vi "Begin.vi"(8 "error in":errorcluster) -> (0 "error out":errorcluster)   [LabVIEW 2016]
doc: "Called before other user functions, this VI is expected to open initial I/O refnums, load in file data, and do all program initialization. Notice that the <B>error out</B> terminal is simply used for data flow. Wiring it to other structures or subVIs ensures that this VI runs first."
uses:
  <vilib>/Rock Robotics/SystemInterfaces/spilib/spi_bus.ctl
  <vilib>/Rock Robotics/WPI/SPI/WPI_SPIMode.ctl
  <vilib>/Rock Robotics/SystemInterfaces/DIO/FPGA_DIOPWMChannel.ctl
  <vilib>/Rock Robotics/WPI/SafetyOutput/WPI_SafetyOutputConfigMenu.ctl
  <vilib>/Rock Robotics/WPI/DriverStation/WPI_DriverStationRobotMode2.ctl
  <vilib>/Rock Robotics/WPI/Joystick/WPI_JoystickDeviceEnum.ctl
  <vilib>/Rock Robotics/SystemInterfaces/DIO/FPGA_DIOChannel.ctl
  <vilib>/Rock Robotics/WPI/Encoder/WPI_EncoderType.ctl
  NI WPI/WPI_SerialPort_USB.ctl
  <vilib>/Rock Robotics/WPI/ThirdParty/CanMotor/TalonSRX/WPI_CANTalonSRX_APIControlMode.ctl
  <vilib>/Rock Robotics/WPI/Solenoid/WPI_SolenoidChannel.ctl
  <vilib>/Rock Robotics/SystemInterfaces/i2clib/i2c_bus.ctl
  <vilib>/Rock Robotics/WPI/Solenoid/WPI_SolenoidValue.ctl
  Robot Global Data.vi
  <vilib>/Rock Robotics/Network Tables/NT Write String Array.vi
  <vilib>/Rock Robotics/WPI/Counter/WPI_CounterDigitalInputToDigitalSource.vi
  navX Library v2/IO/Open/Z900_navX_Open_Serial.vi
  <vilib>/Rock Robotics/WPI/Solenoid/WPI_SolenoidOpenSingle.vi
  <vilib>/Rock Robotics/WPI/MotorControl/WPI_MotorControlOpen VictorSP.vi
  <vilib>/Rock Robotics/WPI/RobotDrive/WPI_RobotDriveOpen4MotorWithVictorSP.vi
  <vilib>/Rock Robotics/WPI/Solenoid/WPI_SolenoidSetEnum.vi
  navX Library v2/navX Library v2.lvlib
  NI WPI/NI WPI Serial USB.lvlib
panel:
  in  "Chip Select Active High (F)":bool
  in  "Mode (3)":T1=enum."Mode 3 (Clk Idle High,Sample on Trailing)"
  in  "Clock Rate (Hz)":dbl=500000.0
  in  "SPI Bus":T2=enum."SPI On-Board, CS1"
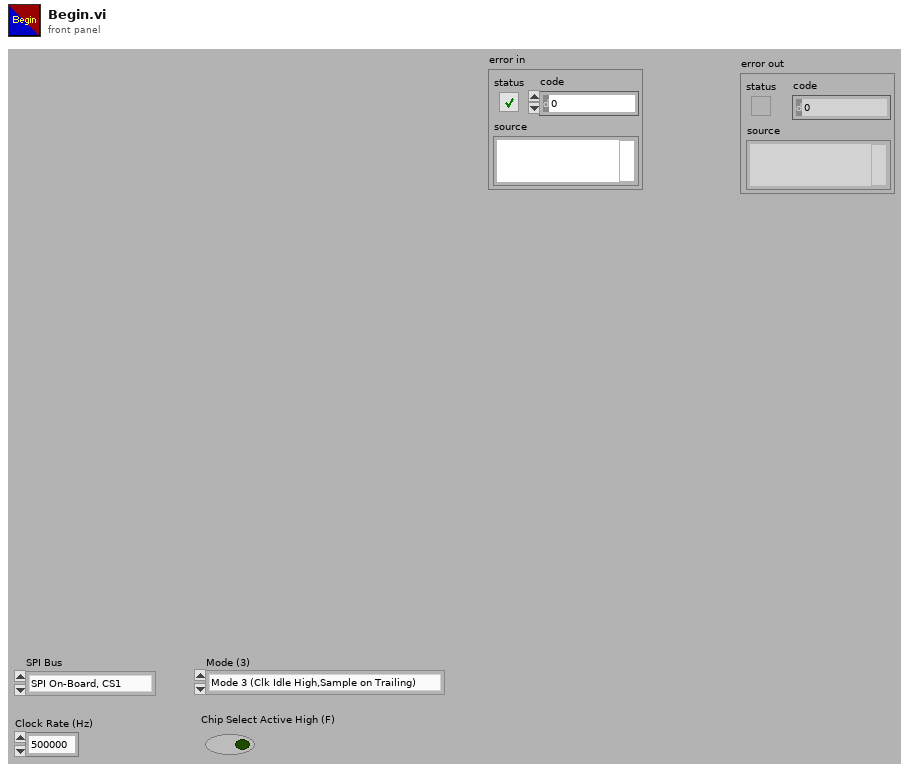
[diagram p1: front panel]
types:
  T1 = typedef "WPI_SPIMode.ctl" = enum16{"Mode 0 (Clk Idle Low,Sample on Leading)", "Mode 1 (Clk Idle Low,Sample on Trailing)", "Mode 2 (Clk Idle High,Sample on Leading)", "Mode 3 (Clk Idle High,Sample on Trailing)"}
  T2 = typedef "spi_bus.ctl" = enum16{"SPI On-Board, CS0", "SPI On-Board, CS1", "SPI On-Board, CS2", "SPI On-Board, CS3", "SPI MXP", "Invalid"}
  T3 = typedef "WPI_CANTalonSRX_APIControlMode.ctl" = enum8{"Percent VBus", "Speed", "Position", "Slave", "Unchanged / Invalid", "Voltage Compensation", "Current", "Motion Profile", "Motion Magic"}
  T4 = typedef "FPGA_DIOPWMChannel.ctl" = enum8{"PWM 0", "PWM 1", "PWM 2", "PWM 3", "PWM 4", "PWM 5", "PWM 6", "PWM 7", "PWM 8", "PWM 9", "PWM MXP 0", "PWM MXP 1", "PWM MXP 2", "PWM MXP 3", "PWM MXP 4", "PWM MXP 5", "PWM MXP 6", "PWM MXP 7", "PWM MXP 8", "PWM MXP 9", "Invalid"}
  T5 = typedef "WPI_SolenoidValue.ctl" = enum16{"Off", "On", "Forward", "Reverse"}
  T6 = typedef "WPI_SolenoidChannel.ctl" = enum8{"Solenoid 0", "Solenoid 1", "Solenoid 2", "Solenoid 3", "Solenoid 4", "Solenoid 5", "Solenoid 6", "Solenoid 7", "Invalid"}
  T7 = typedef "FPGA_DIOChannel.ctl" = enum8{"DIO 0", "DIO 1", "DIO 2", "DIO 3", "DIO 4", "DIO 5", "DIO 6", "DIO 7", "DIO 8", "DIO 9", "DIO MXP 0", "DIO MXP 1", "DIO MXP 2", "DIO MXP 3", "DIO MXP 4", "DIO MXP 5", "DIO MXP 6", "DIO MXP 7", "DIO MXP 8", "DIO MXP 9", "DIO MXP 10", "DIO MXP 11", "DIO MXP 12", "DIO MXP 13", "DIO MXP 14", "DIO MXP 15", "SPI Port CS1", "SPI Port CS2", "SPI Port CS3", "SPI Port MISO", "SPI Port MOSI", "Invalid"}
  T8 = typedef "i2c_bus.ctl" = enum16{"I2C On-Board", "I2C MXP", "Invalid"}
  T9 = typedef "WPI_JoystickDeviceEnum.ctl" = enum16{"USB 0", "USB 1", "USB 2", "USB 3", "USB 4", "USB 5"}
  T10 = typedef "NI WPI Serial USB.lvlib/WPI_SerialPort_USB.ctl" = enum16{"Onboard RS-232", "MXP TTL", "USB"}
  T11 = typedef "WPI_EncoderType.ctl" = enum16{"1x", "2x", "4x"}
  T12 = typedef "WPI_DriverStationRobotMode2.ctl" = enum16{"Autonomous Disabled", "Autonomous Enabled", "Teleop Disabled", "Teleop Enabled", "Disconnected", "Finish", "Test Disabled", "Test Enabled", "Emergency Stopped"}
  T13 = typedef "WPI_SafetyOutputConfigMenu.ctl" = enum16{"Enable", "Disable"}
  T14 = typedef "WPI_JoystickDevRef.ctl" = cluster{"Device":T9}
  T15 = typedef "WPI_I2CDevRef.ctl" = cluster{"DevStatus":errorcluster, "Device Address":u8, "Handle":i32, "I2C Bus":T8}
  T16 = typedef "WPI_MotorControlDeviceRef.ctl" = cluster{"DeviceStatus":errorcluster, "Type":T17, "PWM":cluster{"PWM Channel":T4, "DeadBand":T18}, "CAN":cluster{"Device Number":u8, "SetOutput VI Ref":variant, "GetOutput VI Ref":variant, "Enable VI Ref":variant, "Disable VI Ref":variant, "Data":variant}, "Invert":bool}
  T17 = typedef "WPI_MotorControlType.ctl" = enum16{"PWM", "CAN"}
  T18 = typedef "WPI_PWMDeadband.ctl" = cluster{"Name":string, "maxPositivePwm":i32, "minPositivePwm":i32, "centerPwm":i32, "maxNegativePwm":i32, "minNegativePwm":i32, "angularRange":u16}
  T19 = typedef "WPI_RobotDriveDevRef.ctl" = cluster{"DevStatus":errorcluster, "Motors[]":T16[], "Square Inputs":bool, "Max Output":dbl}
  T20 = typedef "WPI_SPIDevRef.ctl" = cluster{"DevStatus":errorcluster, "Handle":i32, "SPI Bus":T2}
  T21 = typedef "WPI_DigitalInputDevRef.ctl" = cluster{"DevStatus":errorcluster, "DIO Channel":T7}
  T22 = typedef "FPGA_CounterEncoderSourceConvertionLVSourceType.ctl" = cluster{"DevStatus":errorcluster, "AnalogTriggerMode?":bool, "DigitalMode":cluster{"DIO Channel":T23}, "AnalogTriggerMode":cluster{"AnalogTriggerIndex":T24, "OutputType":T25}}
  T23 = typedef "FPGA_DIODigitalSourceChannel.ctl" = enum8{"DIO 0", "DIO 1", "DIO 2", "DIO 3", "DIO 4", "DIO 5", "DIO 6", "DIO 7", "DIO 8", "DIO 9", "DIO MXP 0", "DIO MXP 1", "DIO MXP 2", "DIO MXP 3", "DIO MXP 4", "DIO MXP 5", "DIO MXP 6", "DIO MXP 7", "DIO MXP 8", "DIO MXP 9", "DIO MXP 10", "DIO MXP 11", "DIO MXP 12", "DIO MXP 13", "DIO MXP 14", "DIO MXP 15", "Disabled"}
  T24 = typedef "FPGA_AnalogTriggerIndex.ctl" = enum8{"Trig 0", "Trig 1", "Trig 2", "Trig 3", "Trig 4", "Trig 5", "Trig 6", "Trig 7", "Invalid"}
  T25 = typedef "FPGA_AnalogTriggerOutType.ctl" = enum16{"InWindow", "TriggerState", "Rising", "Falling"}
  T26 = typedef "WPI_EncoderDevRef.ctl" = cluster{"DevStatus":errorcluster, "EncoderIndex":T27, "CounterIndex":T28, "DistancePerCount":dbl, "Decoding Type":T11}
  T27 = typedef "FPGA_EncoderIdx.ctl" = enum8{"Enc 0", "Enc 1", "Enc 2", "Enc 3", "Enc 4", "Enc 5", "Enc 6", "Enc 7", "Invalid"}
  T28 = typedef "FPGA_CounterCtrSystemIndex.ctl" = enum8{"Ctr 0", "Ctr 1", "Ctr 2", "Ctr 3", "Ctr 4", "Ctr 5", "Ctr 6", "Ctr 7", "Invalid"}
  T29 = typedef "navX Library v2.lvlib/Z900_navX_DeviceTypeDef.ctl" = cluster{"Interface":cluster{"Protocol":T30, "Update Rate (4Hz-100Hz)":u8, "navX Open TypeDef":variant}, "Notify Packet":refnum<notifier>, "Loop VI Refnum":refnum<vi>, "Ready to Close Occurrence Refnum":refnum<k4>}
  T30 = typedef "navX Library v2.lvlib/Z900_navX_ProtocolTypeDef.ctl" = enum16{"SERIAL", "I2C", "SPI"}
  T31 = typedef "WPI_SolenoidDevRef.ctl" = cluster{"DevStatus":errorcluster, "Pneumatics Control Module":u8, "Forward Solenoid Channel":T6, "Reverse Solenoid Channel":T6}
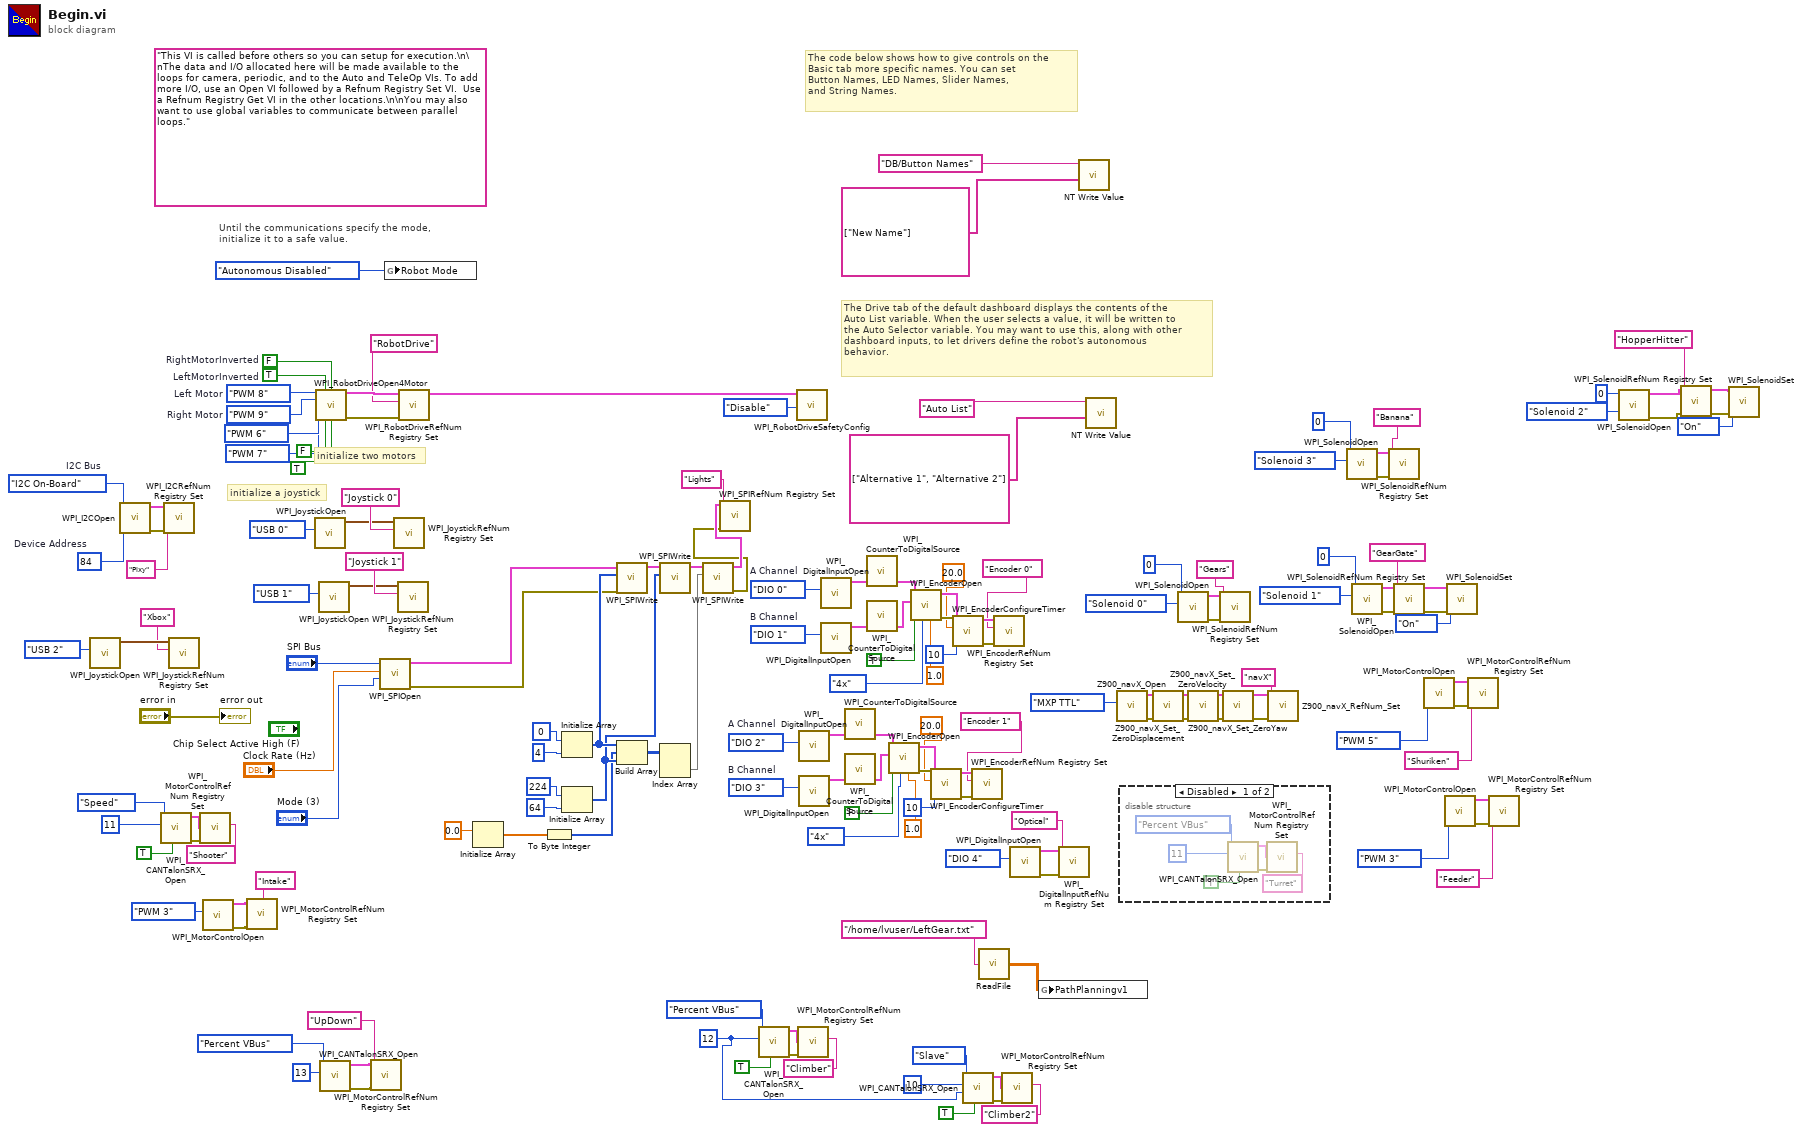
[diagram p0: block diagram]
diagram:
  w59 = u8 84  # Device Address
  w60 = i2c_bus."I2C On-Board"  # I2C Bus
  w18 = 12
  w126 = FPGA_DIOChannel."DIO 3"  # B Channel
  w125 = FPGA_DIOChannel."DIO 2"  # A Channel
  w142 = FPGA_DIOChannel."DIO 1"  # B Channel
  w141 = FPGA_DIOChannel."DIO 0"  # A Channel
  (unwired) "This VI is called before others so you can setup for execution.\n\nThe data and I/O allocated here will be made available to the loops for camera, periodic, and to the Auto and TeleOp VIs. To add more I/O, use an Open VI followed by a Refnum Registry Set VI.  Use a Refnum Registry Get VI in the other locations.\n\nYou may also want to use global variables to communicate between parallel loops."
  w157 = FPGA_DIOPWMChannel."PWM 9"  # Right Motor
  w158 = FPGA_DIOPWMChannel."PWM 8"  # Left Motor
  w162 = TRUE  # LeftMotorInverted
  w163 = FALSE  # RightMotorInverted
  # "The Drive tab of the default dashboard displays the contents of the\nAuto List variable. When the user selects a value, it will be written to\nthe Auto Selector variable. You may want to use this, along with other\ndashboard inputs, to let drivers define the robot's autonomous\nbehavior."
  # "The code below shows how to give controls on the\nBasic tab more specific names. You can set\nButton Names, LED Names, Slider Names,\nand String Names."
  # "initialize a joystick"
  # "Until the communications specify the mode,\ninitialize it to a safe value."
  # "initialize two motors"
  n1 = call <vilib>:"WPI_JoystickOpen.vi"("JoystickDevice"=WPI_JoystickDeviceEnum."USB 2") -> ("JoystickDevRef"=w73:T14)  [unwired: 10 in]
  n2 = call <vilib>:"WPI_I2COpen.vi"("Device Address"=w59, "I2C Bus"=w60) -> ("error out"=w58:errorcluster, "I2CDevRef"=w57:T15)  [unwired: 8 in]
  n3 = call <vilib>:"WPI_CANTalonSRX_Open.vi"("Invert"=TRUE, "Device Number"=11, "Control Mode"=WPI_CANTalonSRX_APIControlMode."Speed") -> ("error out"=w93:errorcluster, "CAN Talon SRX Ref"=w94:T16)  [unwired: 7 in]
  n4 = call <vilib>:"WPI_I2CRefNum Registry Set.vi"("error in (no error)"=w58, "refnum name"="Pixy", "I2CDevRef"=w57) -> ()  [unwired: 7 in, 2 out]
  n5 = call <vilib>:"WPI_JoystickRefNum Registry Set.vi"("refnum name"="Xbox", "JoystickDevRef"=w73) -> ()  [unwired: 8 in, 2 out]
  n6 = call <vilib>:"WPI_MotorControlRefNum Registry Set.vi"("error in (no error)"=w93, "refnum name"="Shooter", "MotorControlDevRef"=w94) -> ()  [unwired: 7 in, 2 out]
  n7 = call-poly <vilib>:"WPI_MotorControlOpen.vi"("PWM Channel"=FPGA_DIOPWMChannel."PWM 3") -> ("error out"=w8:errorcluster, "MotorControlDeviceRef"=w9:T16)  [unwired: 9 in]
  n8 = call <vilib>:"WPI_MotorControlRefNum Registry Set.vi"("error in (no error)"=w8, "refnum name"="Intake", "MotorControlDevRef"=w9) -> ()  [unwired: 7 in, 2 out]
  n9 = call <vilib>:"WPI_JoystickOpen.vi"("JoystickDevice"=WPI_JoystickDeviceEnum."USB 0") -> ("JoystickDevRef"=w152:T14)  [unwired: 10 in]
  n10 = call-poly <vilib>:"WPI_RobotDriveOpen4Motor.vi"("Rear Left Motor"=w158, "Rear Left Motor Inverted"=w162, "Rear Right Motor Inverted"=w163, "Rear Right Motor"=w157, "Front Left Motor"=FPGA_DIOPWMChannel."PWM 6", "Front Right Motor"=FPGA_DIOPWMChannel."PWM 7", "Front Left Motor Inverted"=TRUE, "Front Right Motor Inverted"=FALSE) -> ("RobotDriveDevRef"=w161:T19, "error out"=w159:errorcluster)  [unwired: 6 in]
  n11 = call <vilib>:"WPI_JoystickOpen.vi"("JoystickDevice"=WPI_JoystickDeviceEnum."USB 1") -> ("JoystickDevRef"=w144:T14)  [unwired: 10 in]
  n12 = call <vilib>:"WPI_CANTalonSRX_Open.vi"("Device Number"=u8 13, "Control Mode"=WPI_CANTalonSRX_APIControlMode."Percent VBus") -> ("error out"=w6:errorcluster, "CAN Talon SRX Ref"=w7:T16)  [unwired: 8 in]
  n13 = call <vilib>:"WPI_MotorControlRefNum Registry Set.vi"("error in (no error)"=w6, "refnum name"="UpDown", "MotorControlDevRef"=w7) -> ()  [unwired: 7 in, 2 out]
  n14 = call <vilib>:"WPI_SPIOpen.vi"("Mode (3)"="Mode (3)", "Clock Rate (Hz)"="Clock Rate (Hz)", "SPI Bus"="SPI Bus") -> ("error out"=w28:errorcluster, "SPIDevRef"=w29:T20)  [unwired: 7 in]
  n15 = global write "Robot Global Data.vi" "Robot Mode"(WPI_DriverStationRobotMode2."Autonomous Disabled" ("Robot Mode")) -> ()
  n16 = call <vilib>:"WPI_JoystickRefNum Registry Set.vi"("refnum name"="Joystick 0", "JoystickDevRef"=w152) -> ()  [unwired: 8 in, 2 out]
  n17 = call <vilib>:"WPI_JoystickRefNum Registry Set.vi"("refnum name"="Joystick 1", "JoystickDevRef"=w144) -> ()  [unwired: 8 in, 2 out]
  n18 = call <vilib>:"WPI_RobotDriveRefNum Registry Set.vi"("error in (no error)"=w159, "refnum name"="RobotDrive", "RobotDriveDevRef"=w161) -> ("RobotDriveDevRef"=w156:T19)  [unwired: 1 in, 7 out]
  n19 = Initialize Array(0.0 ("element")) -> (w33:dbl[])  [unwired: 1 in]
  n20 = To Byte Integer(number=w33) -> (8bit integer=w32:i8[])
  n21 = Initialize Array(u8 0 ("Data To Send"), u8 4 ("dimension size")) -> (w37:u8[])
  n22 = Initialize Array(u8 224 ("Data To Send"), u8 64 ("dimension size")) -> (w36:u8[])
  n23 = call <vilib>:"WPI_SPIWrite.vi"("error in (no error)"=w28, "Data To Send"=w37, "SPIDevRef"=w29) -> ("SPIDevRef"=w38:T20)  [unwired: 6 in, 2 out]
  n24 = Build Array(w37, w32, w36) -> (w31:u8[][])
  n25 = call <vilib>:"WPI_SPIWrite.vi"("Data To Send"=w36, "SPIDevRef"=w38) -> ("SPIDevRef"=w35:T20)  [unwired: 7 in, 2 out]
  n26 = Index Array(array=w31) -> (element=w30:u8[])  [unwired: 2 in]
  n27 = call <vilib>:"WPI_SPIWrite.vi"("Data To Send"=w30, "SPIDevRef"=w35) -> ("error out"=w25:errorcluster, "SPIDevRef"=w26:T20)  [unwired: 7 in, 1 out]
  n28 = call <vilib>:"WPI_SPIRefNum Registry Set.vi"("error in (no error)"=w25, "refnum name"="Lights", "SPIDevRef"=w26) -> ()  [unwired: 7 in, 2 out]
  n29 = call <vilib>:"WPI_CANTalonSRX_Open.vi"("Invert"=TRUE, "Device Number"=w18, "Control Mode"=WPI_CANTalonSRX_APIControlMode."Percent VBus") -> ("error out"=w88:errorcluster, "CAN Talon SRX Ref"=w89:T16)  [unwired: 7 in]
  n30 = call <vilib>:"WPI_RobotDriveSafetyConfig.vi"("mode"=WPI_SafetyOutputConfigMenu."Disable", "RobotDriveDevRef"=w156) -> ()  [unwired: 8 in, 2 out]
  n31 = call <vilib>:"WPI_MotorControlRefNum Registry Set.vi"("error in (no error)"=w88, "refnum name"="Climber", "MotorControlDevRef"=w89) -> ()  [unwired: 7 in, 2 out]
  n32 = call <vilib>:"WPI_DigitalInputOpen.vi"("DIO Channel"=w125) -> ("DigitalInputDevRef"=w122:T21)  [unwired: 1 in, 9 out]
  n33 = call <vilib>:"WPI_DigitalInputOpen.vi"("DIO Channel"=w126) -> ("DigitalInputDevRef"=w123:T21)  [unwired: 1 in, 9 out]
  n34 = call <vilib>:"WPI_DigitalInputOpen.vi"("DIO Channel"=w141) -> ("DigitalInputDevRef"=w138:T21)  [unwired: 1 in, 9 out]
  n35 = call <vilib>:"WPI_DigitalInputOpen.vi"("DIO Channel"=w142) -> ("DigitalInputDevRef"=w139:T21)  [unwired: 1 in, 9 out]
  n36 = call-poly <vilib>:"WPI_CounterToDigitalSource.vi"("DigitalInputDevRef"=w122) -> ("Digital Source"=w121:T22)  [unwired: 6 out]
  n37 = call-poly <vilib>:"WPI_CounterToDigitalSource.vi"("DigitalInputDevRef"=w123) -> ("Digital Source"=w124:T22)  [unwired: 6 out]
  n38 = call-poly <vilib>:"WPI_CounterToDigitalSource.vi"("DigitalInputDevRef"=w138) -> ("Digital Source"=w137:T22)  [unwired: 6 out]
  n39 = call-poly <vilib>:"WPI_CounterToDigitalSource.vi"("DigitalInputDevRef"=w139) -> ("Digital Source"=w140:T22)  [unwired: 6 out]
  n40 = call <vilib>:"WPI_EncoderOpen.vi"("DistancePerCount"=1.0, "Decoding Type"=WPI_EncoderType."4x", "Invert Direction (False)"=FALSE, "BSource"=w124, "ASource"=w121) -> ("error out"=w119:errorcluster, "EncoderDevRef"=w118:T26)  [unwired: 3 in, 2 out]
  n41 = call <vilib>:"WPI_EncoderOpen.vi"("DistancePerCount"=1.0, "Decoding Type"=WPI_EncoderType."4x", "Invert Direction (False)"=TRUE, "BSource"=w140, "ASource"=w137) -> ("error out"=w133:errorcluster, "EncoderDevRef"=w132:T26)  [unwired: 3 in, 2 out]
  n42 = call <vilib>:"WPI_EncoderConfigureTimer.vi"("error in (no error)"=w119, "Number Samples to Average"=u8 10, "Minimum Rate"=20.0, "EncoderDevRef"=w118) -> ("error out"=w115:errorcluster, "EncoderDevRef"=w114:T26)  [unwired: 6 in]
  n43 = call <vilib>:"WPI_EncoderConfigureTimer.vi"("error in (no error)"=w133, "Number Samples to Average"=u8 10, "Minimum Rate"=20.0, "EncoderDevRef"=w132) -> ("error out"=w129:errorcluster, "EncoderDevRef"=w128:T26)  [unwired: 6 in]
  n44 = call <vilib>:"WPI_CANTalonSRX_Open.vi"("Invert"=TRUE, "Master Device Number"=w18, "Device Number"=10, "Control Mode"=WPI_CANTalonSRX_APIControlMode."Slave") -> ("error out"=w19:errorcluster, "CAN Talon SRX Ref"=w20:T16)  [unwired: 6 in]
  n45 = call <vilib>:"WPI_EncoderRefNum Registry Set.vi"("error in (no error)"=w115, "refnum name"="Encoder 1", "EncoderDevRef"=w114) -> ()  [unwired: 7 in, 2 out]
  n46 = call "ReadFile.vi"("Name"="/home/lvuser/LeftGear.txt") -> ("Array - Numeric"=w53:dbl[][])
  n47 = call <vilib>:"WPI_EncoderRefNum Registry Set.vi"("error in (no error)"=w129, "refnum name"="Encoder 0", "EncoderDevRef"=w128) -> ()  [unwired: 7 in, 2 out]
  n48 = call <vilib>:"WPI_MotorControlRefNum Registry Set.vi"("error in (no error)"=w19, "refnum name"="Climber2", "MotorControlDevRef"=w20) -> ()  [unwired: 7 in, 2 out]
  n49 = call <vilib>:"WPI_DigitalInputOpen.vi"("DIO Channel"=FPGA_DIOChannel."DIO 4") -> ("error out"=w49:errorcluster, "DigitalInputDevRef"=w48:T21)  [unwired: 9 in]
  n50 = global write "Robot Global Data.vi" "PathPlanningv1"(w53) -> ()
  n51 = call <vilib>:"WPI_DigitalInputRefNum Registry Set.vi"("error in (no error)"=w49, "refnum name"="Optical", "DigitalInputDevRef"=w48) -> ()  [unwired: 7 in, 2 out]
  n52 = call-poly <vilib>:"NT Write Value.vi"("String Array"=string[] ["New Name"], "Name"="DB/Button Names") -> ()  [unwired: 9 in, 1 out]
  n53 = call-poly <vilib>:"NT Write Value.vi"("String Array"=string[] ["Alternative 1", "Alternative 2"], "Name"="Auto List") -> ()  [unwired: 9 in, 1 out]
  n54 = call-poly "Z900_navX_Open.vi"("Serial Port"=WPI_SerialPort_USB."MXP TTL") -> ("error out"=w101:errorcluster, "navX Device"=w106:T29)  [unwired: 9 in]
  n55 = disable-structure shown="Disabled" {
    frame Disabled {
      n56 = call <vilib>:"WPI_CANTalonSRX_Open.vi"("Invert"=TRUE, "Device Number"=11, "Control Mode"=WPI_CANTalonSRX_APIControlMode."Percent VBus") -> ("error out"=w164:errorcluster, "CAN Talon SRX Ref"=w165:T16)  [unwired: 7 in]
      n57 = call <vilib>:"WPI_MotorControlRefNum Registry Set.vi"("error in (no error)"=w164, "refnum name"="Turret", "MotorControlDevRef"=w165) -> ()  [unwired: 7 in, 2 out]
    }
    frame Enabled {
    }
  }
  n58 = call "Z900_navX_Set_ZeroDisplacement.vi"("error in (no error)"=w101, "navX Device"=w106) -> ("error out"=w100:errorcluster, "navX Device"=w105:T29)  [unwired: 8 in]
  n59 = call-poly <vilib>:"WPI_SolenoidOpen.vi"("Solenoid Channel"=WPI_SolenoidChannel."Solenoid 0", "Pneumatics Control Module (0)"=u8 0) -> ("error out"=w87:errorcluster, "SolenoidDevRef"=w86:T31)  [unwired: 8 in]
  n60 = call "Z900_navX_Set_ZeroVelocity.vi"("error in (no error)"=w100, "navX Device"=w105) -> ("error out"=w99:errorcluster, "navX Device"=w104:T29)  [unwired: 8 in]
  n61 = call <vilib>:"WPI_SolenoidRefNum Registry Set.vi"("error in (no error)"=w87, "refnum name"="Gears", "SolenoidDevRef"=w86) -> ()  [unwired: 7 in, 2 out]
  n62 = call "Z900_navX_Set_ZeroYaw.vi"("error in (no error)"=w99, "navX Device"=w104) -> ("error out"=w102:errorcluster, "navX Device"=w103:T29)  [unwired: 8 in]
  n63 = call "Z900_navX_RefNum_Set.vi"("error in (no error)"=w102, "refnum name"="navX", "navX Device"=w103) -> ()  [unwired: 7 in, 2 out]
  n64 = call-poly <vilib>:"WPI_SolenoidOpen.vi"("Solenoid Channel"=WPI_SolenoidChannel."Solenoid 3", "Pneumatics Control Module (0)"=u8 0) -> ("error out"=w65:errorcluster, "SolenoidDevRef"=w64:T31)  [unwired: 8 in]
  n65 = call-poly <vilib>:"WPI_SolenoidOpen.vi"("Solenoid Channel"=WPI_SolenoidChannel."Solenoid 1", "Pneumatics Control Module (0)"=u8 0) -> ("error out"=w78:errorcluster, "SolenoidDevRef"=w77:T31)  [unwired: 8 in]
  n66 = call <vilib>:"WPI_SolenoidRefNum Registry Set.vi"("error in (no error)"=w65, "refnum name"="Banana", "SolenoidDevRef"=w64) -> ()  [unwired: 7 in, 2 out]
  n67 = call <vilib>:"WPI_SolenoidRefNum Registry Set.vi"("error in (no error)"=w78, "refnum name"="GearGate", "SolenoidDevRef"=w77) -> ("error out"=w52:errorcluster, "SolenoidDevRef"=w51:T31)  [unwired: 7 in]
  n68 = call-poly <vilib>:"WPI_MotorControlOpen.vi"("PWM Channel"=FPGA_DIOPWMChannel."PWM 5") -> ("error out"=w82:errorcluster, "MotorControlDeviceRef"=w81:T16)  [unwired: 9 in]
  n69 = call-poly <vilib>:"WPI_MotorControlOpen.vi"("PWM Channel"=FPGA_DIOPWMChannel."PWM 3") -> ("error out"=w70:errorcluster, "MotorControlDeviceRef"=w69:T16)  [unwired: 9 in]
  n70 = call-poly <vilib>:"WPI_SolenoidSet.vi"("error in (no error)"=w52, "Value"=WPI_SolenoidValue."On", "SolenoidDevRef"=w51) -> ()  [unwired: 7 in, 2 out]
  n71 = call <vilib>:"WPI_MotorControlRefNum Registry Set.vi"("error in (no error)"=w82, "refnum name"="Shuriken", "MotorControlDevRef"=w81) -> ()  [unwired: 7 in, 2 out]
  n72 = call <vilib>:"WPI_MotorControlRefNum Registry Set.vi"("error in (no error)"=w70, "refnum name"="Feeder", "MotorControlDevRef"=w69) -> ()  [unwired: 7 in, 2 out]
  n73 = call-poly <vilib>:"WPI_SolenoidOpen.vi"("Solenoid Channel"=WPI_SolenoidChannel."Solenoid 2", "Pneumatics Control Module (0)"=u8 0) -> ("error out"=w16:errorcluster, "SolenoidDevRef"=w17:T31)  [unwired: 8 in]
  n74 = call <vilib>:"WPI_SolenoidRefNum Registry Set.vi"("error in (no error)"=w16, "refnum name"="HopperHitter", "SolenoidDevRef"=w17) -> ("error out"=w11:errorcluster, "SolenoidDevRef"=w12:T31)  [unwired: 7 in]
  n75 = call-poly <vilib>:"WPI_SolenoidSet.vi"("error in (no error)"=w11, "Value"=WPI_SolenoidValue."On", "SolenoidDevRef"=w12) -> ()  [unwired: 7 in, 2 out]
  "error out" <- "error in"
